vi "Register for Events.vi"(8 "error in (no error)":errorcluster, 11 "Execution API In":refnum<class "Execution API.lvclass">) -> (0 "error out":errorcluster, 2 "Result Registration Refnum":T1, 3 "Execution API Out":refnum<class "Execution API.lvclass">)   [LabVIEW 2020, in "Execution API.lvclass"]
doc: "Obtain an event registration which can be used to observe the execution while running and obtain results."
uses:
  Execution API.lvclass
  Result Types/Method Result/Method Result.ctl
  Result Types/Assertion Result/Public/TypeDefs/Status.ctl
  Result Types/Assertion Result/Assertion Result.ctl
  Result Types/Assertion Result/Public/TypeDefs/Assertion Type.ctl
  Result Types/Case Result/Test Case Result.ctl
  Result Types/Suite Results/Test Suite Result.ctl
  Execution API.lvclass/Execution API.ctl
  Test Runner/Test Runner.lvclass/Test Runner.ctl
  Result Collector/Result Collector.lvclass/Result Collector.ctl
  Result Collector/Result Collector.lvclass
  Test Runner/Test Runner.lvclass
  Result Types/Assertion Result/Assertion Result.lvlib
  Result Types/Method Result/Method Result.lvlib
  Result Types/Case Result/Test Case Result.lvlib
  Result Types/Suite Results/Test Suite Result.lvlib
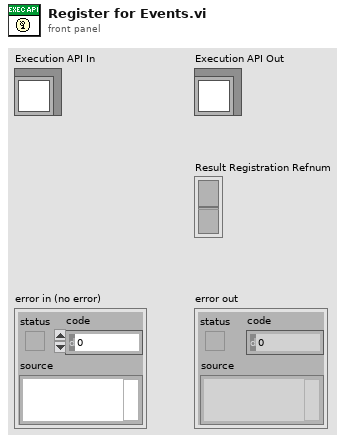
[diagram p1: front panel]
types:
  T1 = cluster{"Result Events":refnum<event-registration>, "Event Registration Refnum":refnum<event-registration>}
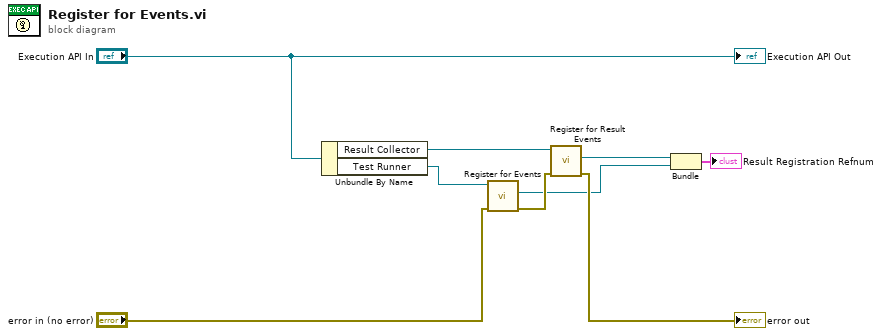
[diagram p0: block diagram]
diagram:
  n1 = Unbundle By Name("Execution API In") -> ("Result Collector"=w8:refnum<class "Result Collector.lvclass">, "Test Runner"=w7:refnum<class "Test Runner.lvclass">)
  n2 = call "Register for Events.vi"("error in (no error)"="error in (no error)", "Test Runner In"=w7) -> ("error out"=w6:errorcluster, "Event Registration Refnum"=w3:refnum<event-registration>)  [unwired: 7 in, 1 out]
  n3 = call "Register for Result Events.vi"("error in (no error)"=w6, "Result Collector In"=w8) -> ("error out"=→"error out":errorcluster, "Result Events"=w2:refnum<event-registration>)  [unwired: 7 in, 1 out]
  n4 = Bundle("Result Events"=w2, "Event Registration Refnum"=w3) -> (→"Result Registration Refnum":T1)  [unwired: 1 in]
  "Execution API Out" <- "Execution API In"
